vi "Init.vi"(6 "Channels":T2[](array[typedef]), 7 "Group Data Type":T1, 8 "error in (no error)":errorcluster, 9 "Raw Values (T)":bool=TRUE, 10 "Multicast Endpoint (None)":T3, 11 "Group Info":T4) -> (0 "error out":errorcluster, 3 "Group Config out":refnum<class "Group Config.lvclass">)   [LabVIEW 2020, in "VectoConfig.lvlib" / "Group Config.lvclass"]
uses:
  Group Config.lvclass
  Group Info.ctl
  Publish Config.ctl
  Channel Init.ctl
  Group Data Type.ctl
  Group Config.lvclass/Group Config.ctl
  VectoConfig/VectoConfig.lvlib
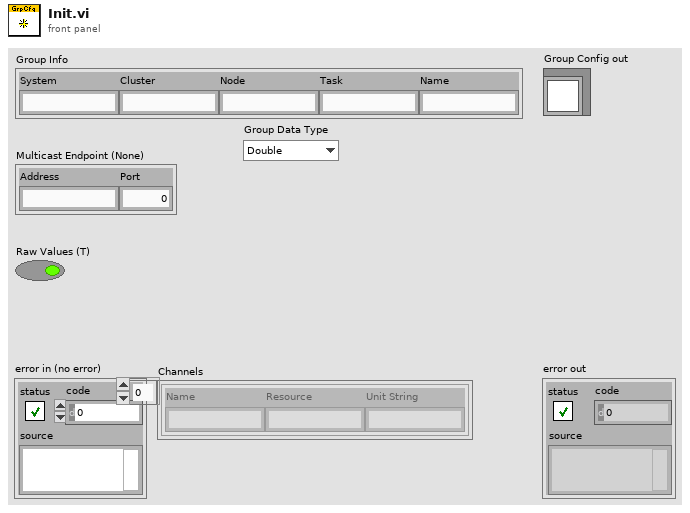
[diagram p1: front panel]
types:
  T1 = typedef "VectoConfig.lvlib/Group Data Type.ctl" = enum16{"Double", "String", "Bool"}
  T2 = typedef "VectoConfig.lvlib/Channel Init.ctl" = cluster{"Name":string, "Resource":string, "Unit String":string}
  T3 = typedef "VectoConfig.lvlib/Publish Config.ctl" = cluster{"Address":string, "Port":u16}
  T4 = typedef "VectoConfig.lvlib/Group Info.ctl" = cluster{"System":string, "Cluster":string, "Node":string, "Task":string, "Name":string}
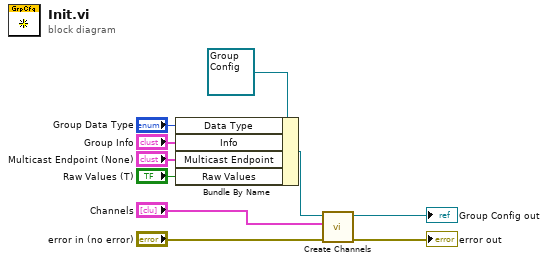
[diagram p0: block diagram]
diagram:
  n1 = Bundle By Name(cluster=refnum<class "Group Config.lvclass"> refnum ("Group Config in"), "Data Type"="Group Data Type", "Info"="Group Info", "Multicast Endpoint"="Multicast Endpoint (None)", "Raw Values"="Raw Values (T)") -> (w4:refnum<class "Group Config.lvclass">)
  n2 = call "Create Channels.vi"("error in (no error)"="error in (no error)", "Channels"="Channels", "Group Config in"=w4) -> ("error out"=→"error out":errorcluster, "Group Config out"=→"Group Config out":refnum<class "Group Config.lvclass">)  [unwired: 7 in]
